vi "ExampleStateMachine-Calculator.vi"() -> ()   [LabVIEW 2018]
panel:
  in  "stop":bool
  in  "CLR":bool
  in  "DIV":bool
  in  "MULT":bool
  in  "SUB":bool
  in  "ADD":bool
  out "Result":dbl
  in  "Number 2":dbl=2.0
  in  "Number 1":dbl=4.0
  # "NOTES:\n\nTurn on Highlight Execution on the Block Diagram before running this program.\n\nSet the numbers to the values you want, and this calculator will compute the sum,\ndifference, product, and quotient of those two numbers when you click on the \ncorresponding buttons."
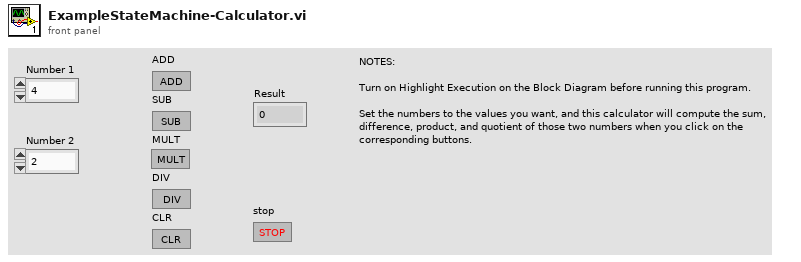
[diagram p1: front panel]
types:
  T1 = enum16{"Wait", "Add", "Subtract", "Multiply", "Divide", "Clear"}
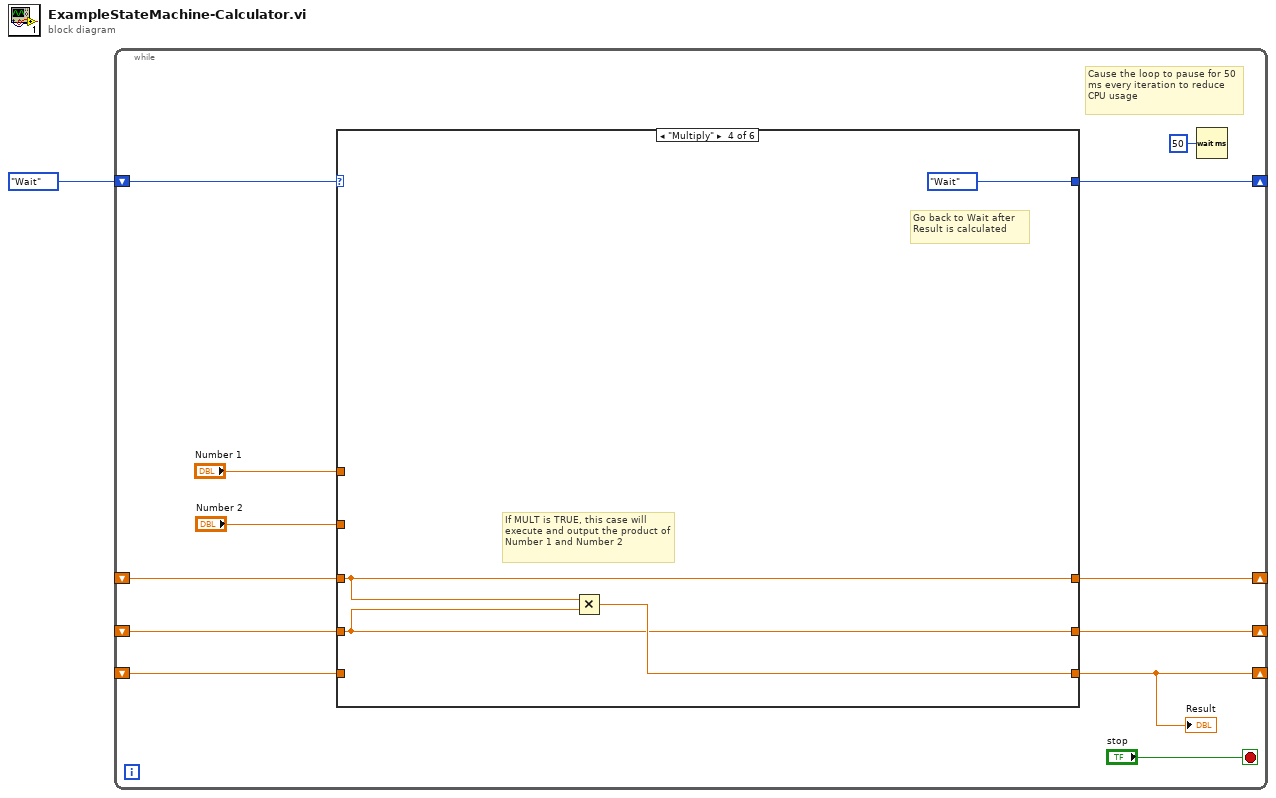
[diagram p0: block diagram]
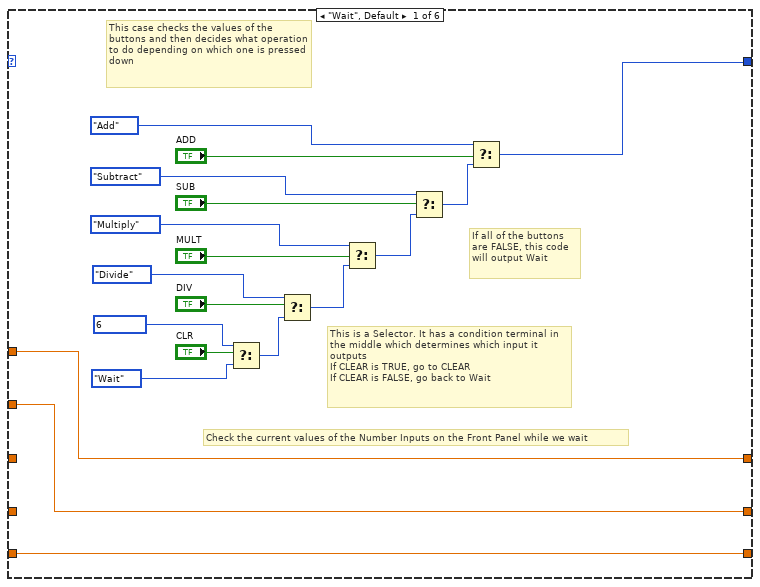
[diagram p2: hidden frame]
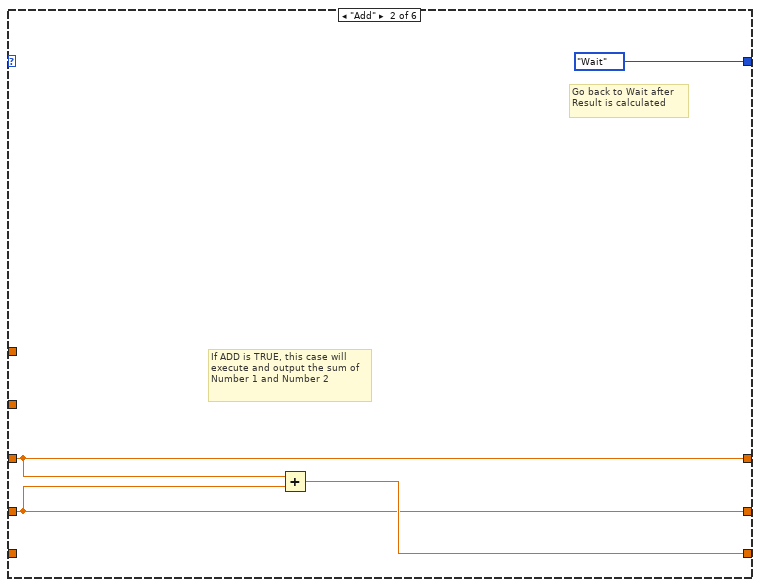
[diagram p3: hidden frame]
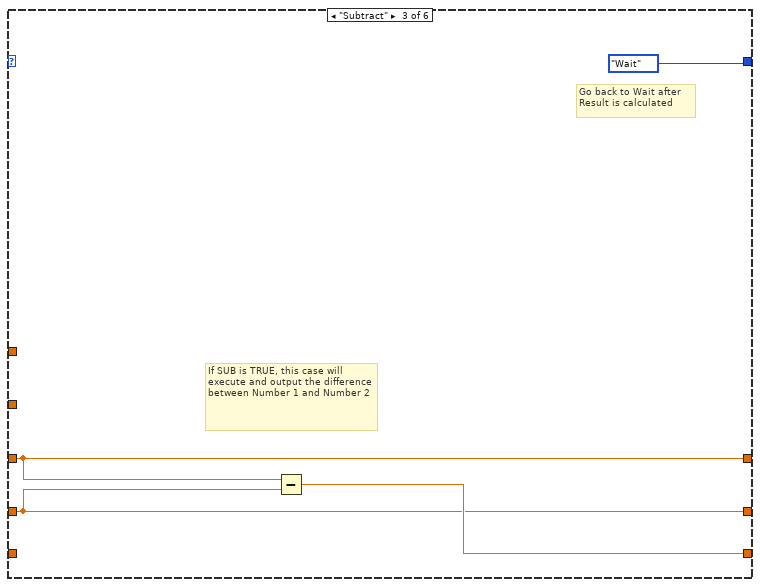
[diagram p4: hidden frame]
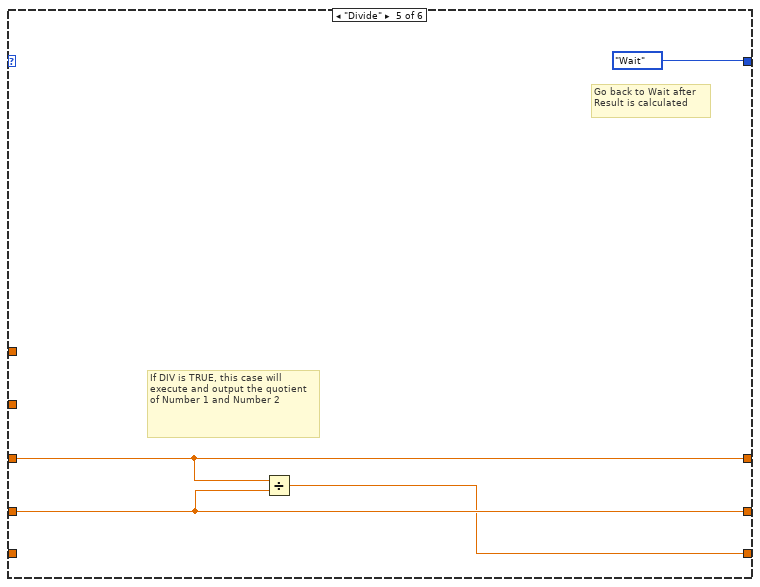
[diagram p5: hidden frame]
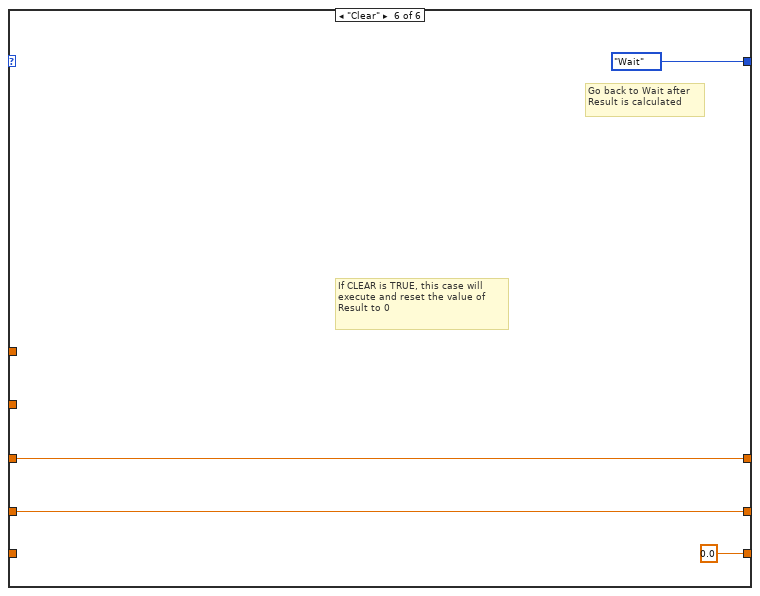
[diagram p6: hidden frame]
diagram:
  n1 = while {
    shift-right: [w12] -> _
    shift-left: _ -> [w8]
    shift-right: [w11] -> _
    shift-left: _ -> [w7]
    shift-right: [w9] -> _
    shift-left: T1."Wait" -> [w13]
    shift-right: [w6] -> _
    shift-left: _ -> [w5]
    stop <- "stop" stop-if-true
    # "Cause the loop to pause for 50 ms every iteration to reduce CPU usage"
    n2 = case shown="\"Multiply\"" w13 {
      tunnel: [w15 w34 w39 w43 w48 w51] -> w12
      tunnel: [w14 w33 w38 w42 w47 w50] -> w11
      tunnel: [w17 T1."Wait" T1."Wait" T1."Wait" T1."Wait" T1."Wait"] -> w9
      tunnel: w8 -> [_ w34 w39 w43 w48 w51]
      tunnel: w7 -> [_ w33 w38 w42 w47 w50]
      tunnel: [w16 w35 w40 w44 w46 0.0] -> w6
      tunnel: w5 -> [w16 _ _ _ _ _]
      tunnel: "Number 1" -> [w15 _ _ _ _ _]
      tunnel: "Number 2" -> [w14 _ _ _ _ _]
      frame "Wait", Default {
        # "Check the current values of the Number Inputs on the Front Panel while we wait"
        # "If all of the buttons are FALSE, this code will output Wait"
        # "This is a Selector. It has a condition terminal in the middle which determines which input it outputs \nIf CLEAR is TRUE, go to CLEAR\nIf CLEAR is FALSE, go back to Wait"
        # "This case checks the values of the buttons and then decides what operation to do depending on which one is pressed down"
        n3 = Select(t=T1 6, s="CLR", f=T1."Wait") -> (s? t:f=w29:T1)
        n4 = Select(t=T1."Divide", s="DIV", f=w29) -> (s? t:f=w27:T1)
        n5 = Select(t=T1."Multiply", s="MULT", f=w27) -> (s? t:f=w25:T1)
        n6 = Select(t=T1."Subtract", s="SUB", f=w25) -> (s? t:f=w23:T1)
        n7 = Select(t=T1."Add", s="ADD", f=w23) -> (s? t:f=w17:T1)
      }
      frame "Add" {
        # "Go back to Wait after Result is calculated"
        # "If ADD is TRUE, this case will execute and output the sum of Number 1 and Number 2"
        n8 = Add(x=w34, y=w33) -> (x+y=w35:dbl)
      }
      frame "Subtract" {
        # "Go back to Wait after Result is calculated"
        # "If SUB is TRUE, this case will execute and output the difference between Number 1 and Number 2"
        n9 = Subtract(x=w39, y=w38) -> (x-y=w40:dbl)
      }
      frame "Multiply" {
        # "If MULT is TRUE, this case will execute and output the product of Number 1 and Number 2"
        # "Go back to Wait after Result is calculated"
        n10 = Multiply(x=w43, y=w42) -> (x*y=w44:dbl)
      }
      frame "Divide" {
        # "If DIV is TRUE, this case will execute and output the quotient of Number 1 and Number 2"
        # "Go back to Wait after Result is calculated"
        n11 = Divide(x=w48, y=w47) -> (x/y=w46:dbl)
      }
      frame "Clear" {
        # "Go back to Wait after Result is calculated"
        # "If CLEAR is TRUE, this case will execute and reset the value of Result to 0"
      }
    }
    "Result" <- w6
    n12 = Wait (ms)(milliseconds to wait=u32 50) -> ()  [unwired: 1 out]
  }
